vi "FTW-Expression-ConstructLexicon.vi"(11 "error in":errorcluster) -> (4 "Compiled Lexer Expression":i64, 6 "Lexicon":string[](array[string]), 8 "Time to Construct":dbl format="%.6fsec", 15 "error out":errorcluster)   [LabVIEW 2013]
uses:
  Regex/FTWLib-PCRE.dll
panel:
  # "Inputs"
  # "Outputs"
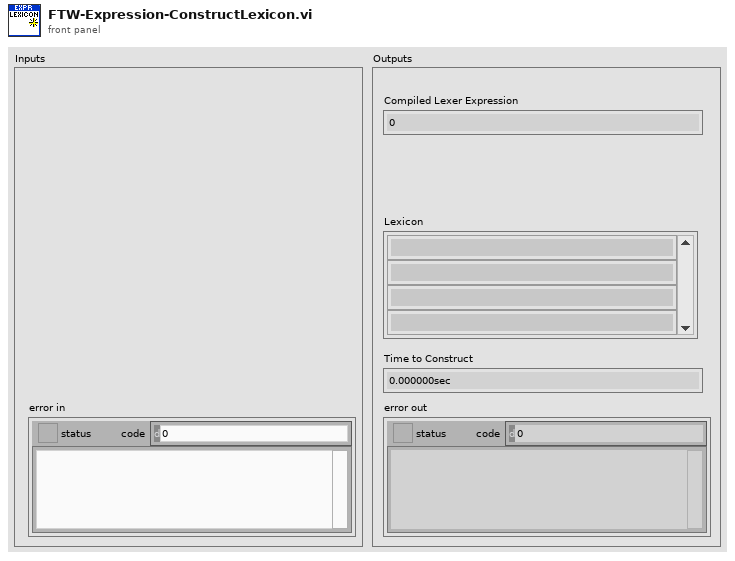
[diagram p1: front panel]
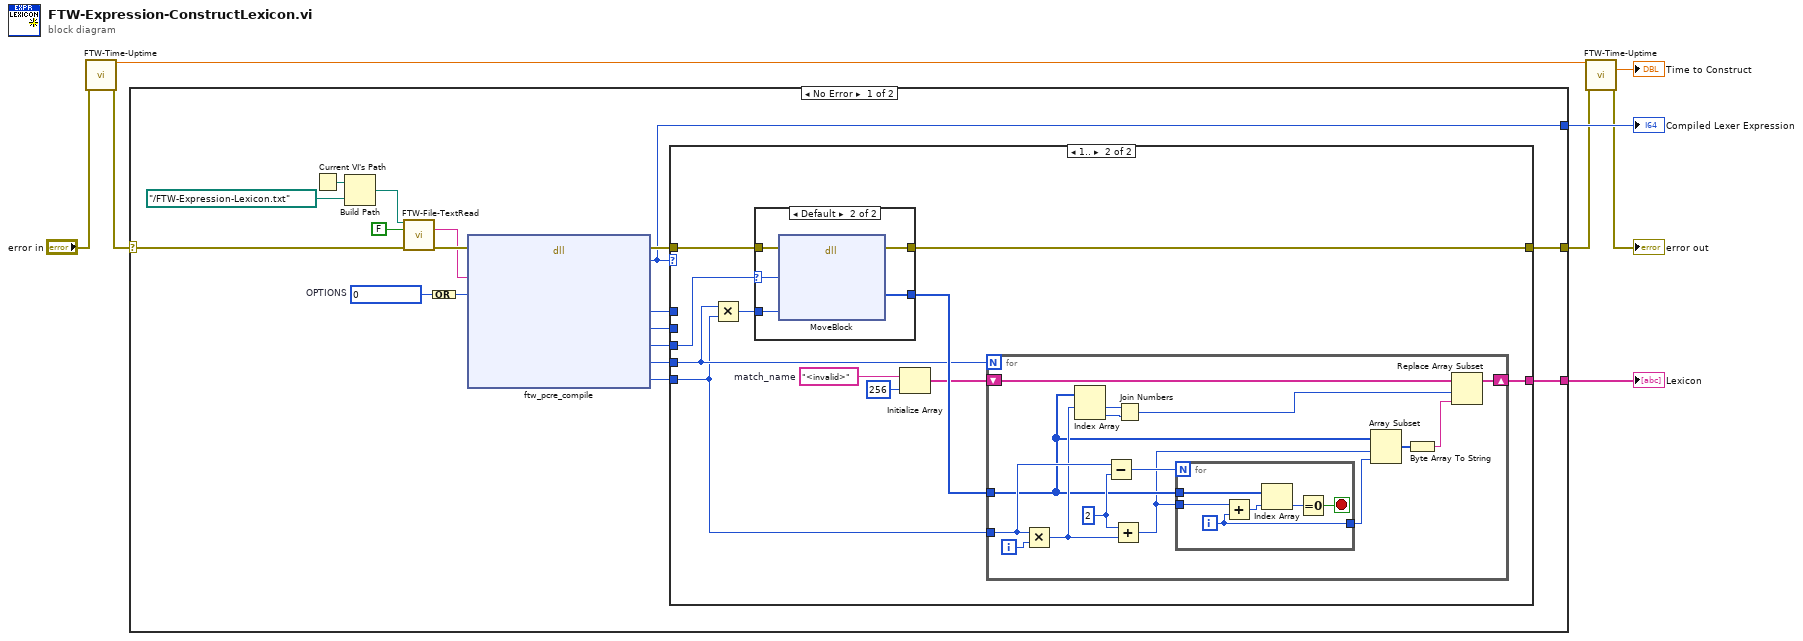
[diagram p0: block diagram]
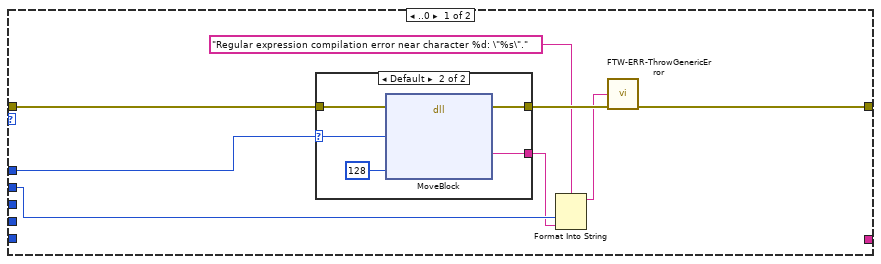
[diagram p2: hidden frame]
diagram:
  n1 = call "FTW-Time-Uptime.vi"("error in"="error in") -> ("Current Uptime"=w2:dbl, "error out"=w7:errorcluster)  [unwired: 12 in, 1 out]
  n2 = case shown="No Error" w7 {
    selector: w7 -> [w23 w79]
    tunnel: [w9 w79] -> w4
    tunnel: [w12 _] -> w6
    tunnel: [w13 _] -> w3
    frame No Error {
      w16 = 0  # OPTIONS
      n3 = Current VI's Path() -> (path=w25:path)
      n4 = Build Path(base path=w25, name or relative path=path "../FTW-Expression-Lexicon.txt" ("path")) -> (appended path=w24:path)
      n5 = call "FTW-File-TextRead.vi"("Filepath"=w24, "Create if doesn't exist?"=FALSE, "error in"=w23) -> ("Text"=w20:string, "error out"=w22:errorcluster)  [unwired: 10 in, 1 out]
      n6 = Compound Arithmetic op=OR(w16) -> (w15:i32)
      n7 = dll-call lib="C:/Users/Jack/repo/ftw-vps/Core/src/Regex/FTWLib-PCRE.*" fn="ftw_pcre_compile"(error in=w22, "Pattern"=w20, "Options"=w15) -> (error out=w14:errorcluster, "PCRE ID"=w12:i64, "Error String"=w11:i64, "Error Offset in Pattern"=w10:i64, "Named Capturing Group Table*"=w19:i64, "Named Capturing Group Count"=w18:i32, "Named Capturing Group Length"=w17:i32)  [unwired: 9 in, 1 out]
      n8 = case shown="1.." w12 {
        tunnel: w19 -> [_ w51]
        tunnel: w18 -> [_ w42]
        tunnel: w17 -> [_ w41]
        tunnel: w14 -> [w34 w46]
        tunnel: [_ w45] -> w13
        tunnel: w11 -> [w33 _]
        tunnel: w10 -> [w30 _]
        tunnel: [w27 w44] -> w9
        frame ..0 {
          n9 = case shown="Default" w33 {
            selector: w33 -> [_ w38]
            tunnel: [_ w40] -> w29
            tunnel: w34 -> [w35 w37]
            tunnel: [w35 w36] -> w32
            frame 0 {
            }
            frame Default {
              n10 = dll-call lib="LabVIEW" fn="MoveBlock"(error in=w37, "Source Pointer"=w38, "Buffer Size"=128 ("dimension size")) -> (error out=w36:errorcluster, "Destination Buffer"=w40:string)  [unwired: 6 in, 1 out]
            }
          }
          n11 = Format Into String(format string="Regular expression compilation error near character %d: \"%s\".", w30, w29) -> (resulting string=w28:string)  [unwired: 2 in, 1 out]
          n12 = call "FTW-ERR-ThrowGenericError.vi"("Error Message"=w28, "error in"=w32) -> ("error out"=w27:errorcluster)  [unwired: 13 in]
        }
        frame 1.. {
          w47 = "<invalid>"  # match_name
          n13 = Multiply(x=w42, y=w41) -> (x*y=w43:i32)
          n14 = case shown="Default" w51 {
            selector: w51 -> [_ w77]
            tunnel: [_ w78] -> w50
            tunnel: w43 -> [_ w76]
            tunnel: w46 -> [w73 w75]
            tunnel: [w73 w74] -> w44
            frame 0 {
            }
            frame Default {
              n15 = dll-call lib="LabVIEW" fn="MoveBlock"(error in=w75, "Source Pointer"=w77, "Buffer Size"=w76) -> (error out=w74:errorcluster, "Destination Buffer"=w78:u8[])  [unwired: 6 in, 1 out]
            }
          }
          n16 = Initialize Array(w47, 256 ("dimension size")) -> (w48:string[])
          n17 = for {
            N: w42 -> [_]
            tunnel: w41 -> [w63]
            tunnel: w50 -> [w59]
            shift-right: [w52] -> w45
            shift-left: w48 -> [w55]
            i -> [w66]
            w61 = 2 ("y")
            n18 = Multiply(x=w63, y=w66) -> (x*y=w60:i32)
            n19 = Index Array(array=w59, index #1=w60) -> (element #1=w65:u8, element #2=w64:u8)  [unwired: 1 in]
            n20 = Subtract(x=w63, y=w61) -> (x-y=w62:i32)
            n21 = Add(x=w61, y=w60) -> (x+y=w56:i32)
            n22 = Join Numbers(hi=w65, lo=w64) -> ((hi.lo)=w54:u16)
            n23 = for {
              N: w62 -> [_]
              tunnel: w59 -> [w72]
              tunnel: w56 -> [w71]
              tunnel: [w67] -> w57
              i -> [w67]
              stop <- w68 stop-if-true
              n24 = Add(x=w71, y=w67) -> (x+y=w70:i32)
              n25 = Index Array(array=w72, index=w70) -> (element=w69:u8)
              n26 = Equal To 0?(x=w69) -> (x = 0?=w68:bool)
            }
            n27 = Array Subset(array=w59, index=w56, length=w57) -> (w58:u8[])
            n28 = Byte Array To String(unsigned byte array=w58) -> (string=w53:string)
            n29 = Replace Array Subset(array=w55, new element=w53, index=w54) -> (w52:string[])
          }
        }
      }
    }
    frame Error {
    }
  }
  "Compiled Lexer Expression" <- w6
  "Lexicon" <- w3
  n30 = call "FTW-Time-Uptime.vi"("Previous Uptime"=w2, "error in"=w4) -> ("Elapsed Time"=→"Time to Construct":dbl, "error out"=→"error out":errorcluster)  [unwired: 11 in, 1 out]
